vi "VA_AoWrite.vi"(4 "error in":errorcluster, 6 "data":dbl[](array[numeric]) format="%0.2f", 7 "task/channels in":refnum<k21>) -> (1 "dataOut":dbl[](array[numeric]) format="%0.2f", 2 "error out":errorcluster, 3 "task out":refnum<k21>)   [LabVIEW 2011]
uses:
  <vilib>/DAQmx/write.llb/DAQmx Write (Analog 1D DBL NChan 1Samp).vi
  <vilib>/DAQmx/miscellaneous.llb/DAQmx Fill In Error Info.vi
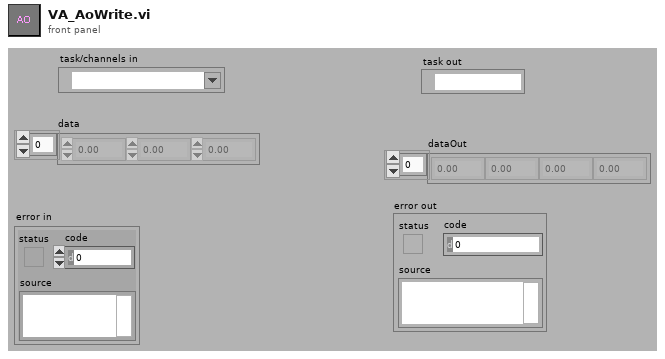
[diagram p1: front panel]
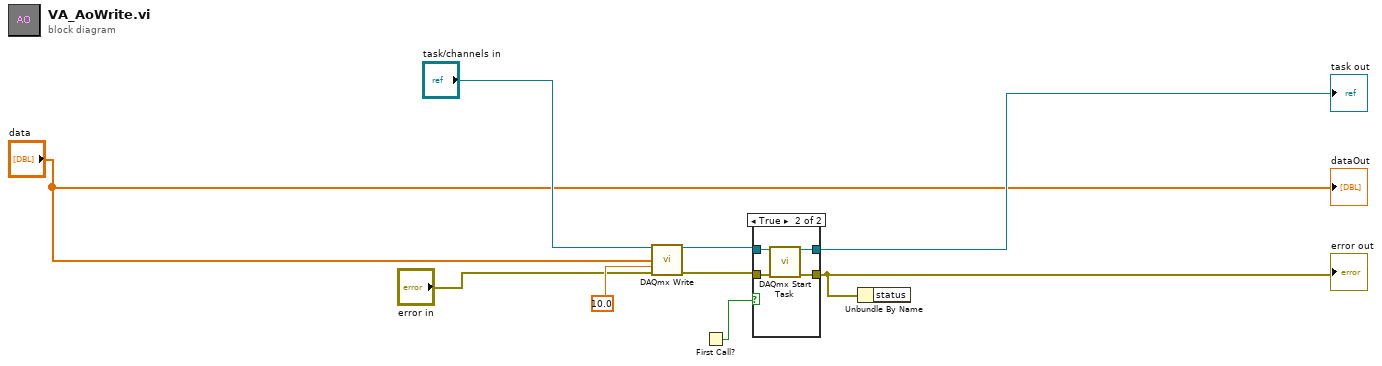
[diagram p0: block diagram]
diagram:
  n1 = call-poly <vilib>:"DAQmx Write.vi"("task/channels in"="task/channels in", "data"="data", "timeout"=10.0, "error in"="error in") -> ("task out"=w7:refnum<k21>, "error out"=w6:errorcluster)  [unwired: 9 in, 1 out]
  n2 = First Call?() -> (First Call?: T/F=w8:bool)
  n3 = case shown="True" w8 {
    tunnel: w7 -> [w11 w15]
    tunnel: w6 -> [w10 w14]
    tunnel: [w10 w13] -> w4
    tunnel: [w11 w12] -> w5
    frame False {
      # "7b."
    }
    frame True {
      n4 = call <vilib>:"DAQmx Start Task.vi"("task/channels in"=w15, "error in"=w14) -> ("task out"=w12:refnum<k21>, "error out"=w13:errorcluster)  [unwired: 12 in]
    }
  }
  "task out" <- w5
  "error out" <- w4
  n5 = Unbundle By Name(w4) -> ()  [unwired: 1 out]
  "dataOut" <- "data"
